vi "Bitwise NOT (Greyscale with Mask).vi"(8 "error in (no error)":errorcluster, 9 "Mask in":T1, 10 "Greyscale Image Destination in":T1, 11 "Greyscale Image Source in":T1) -> (0 "error out":errorcluster, 3 "Greyscale Image Destination":T1)   [LabVIEW 2020, in "image.lvlib"]
doc: "Compute the bitwise NOT of the pixels in the Source Image with a mask."
uses:
  image.lvlib
  Greyscale Image.ctl
  f9ee80d6-438b-4cfb-91f1-04b98ac80474.vi
  <vilib>/Utility/error.llb/Error Cluster From Error Code.vi
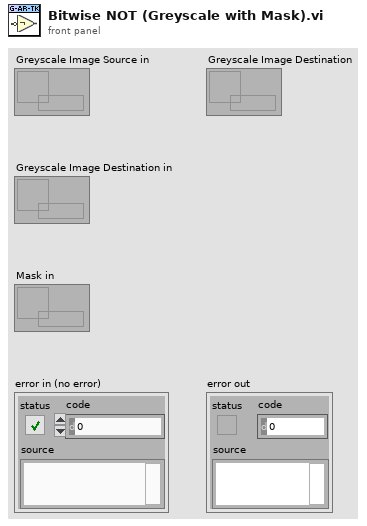
[diagram p1: front panel]
types:
  T1 = typedef "image.lvlib/Greyscale Image.ctl" = refnum<data-value>
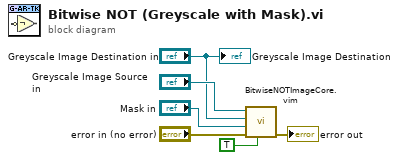
[diagram p0: block diagram]
diagram:
  n1 = call "BitwiseNOTImageCore.vim"("HasMask"=TRUE, "error in (no error)"="error in (no error)", "Mask"="Mask in", "Greyscale Image Destination"="Greyscale Image Destination in", "Greyscale Image Source"="Greyscale Image Source in") -> ("error out"=→"error out":errorcluster)  [unwired: 6 in]
  "Greyscale Image Destination" <- "Greyscale Image Destination in"
